vi "picoharp_start_stream.vi"(8 "error in (no error)":errorcluster, 11 "hydraharp in":refnum<class "picoharp.lvclass">) -> (0 "error out":errorcluster, 3 "hydraharp out":refnum<class "picoharp.lvclass">)   [LabVIEW 2015, in "picoharp.lvclass"]
uses:
  picoharp.lvclass
  picoharp.lvclass/picoharp.ctl
  Hydraharp/hydraharp/hydraharp_fifo_queue_data.ctl
  Hydraharp/hydraharp/hydraharp_fifo_actions.ctl
  Hydraharp/raw_stream_logger/raw_stream_logger.lvclass
  Hydraharp/hdf5_photon_record_logger/hdf5_photon_record_log.lvclass
  Data Logger Class/data_logger.lvclass
  phlib.dll
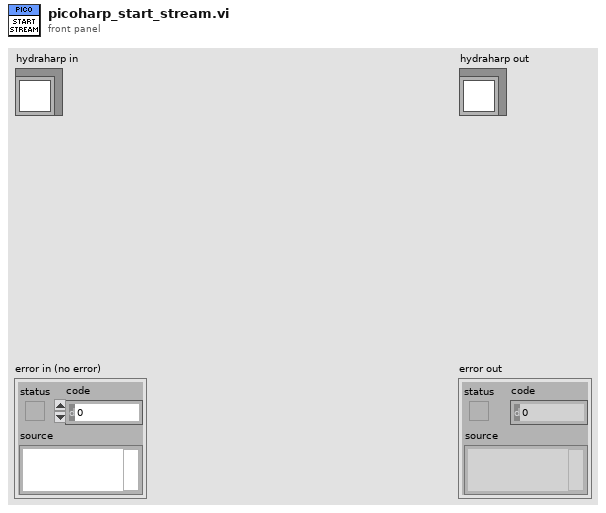
[diagram p1: front panel]
types:
  T1 = typedef "hydraharp_fifo_queue_data.ctl" = cluster{"fifo_buffer":u32[], "fifo_action":T2}
  T2 = typedef "hydraharp_fifo_actions.ctl" = enum16{"stop", "new_data"}
  T3 = typedef "hydraharp_action_on_records.ctl" = enum16{"stream_to_file", "correlate", "stream to file and correlate"}
  T4 = typedef "hpanel_acq_modes.ctl" = u16
  T5 = typedef "record_type.ctl" = enum16{"Raw Stream", "Processed Records (hdf5)"}
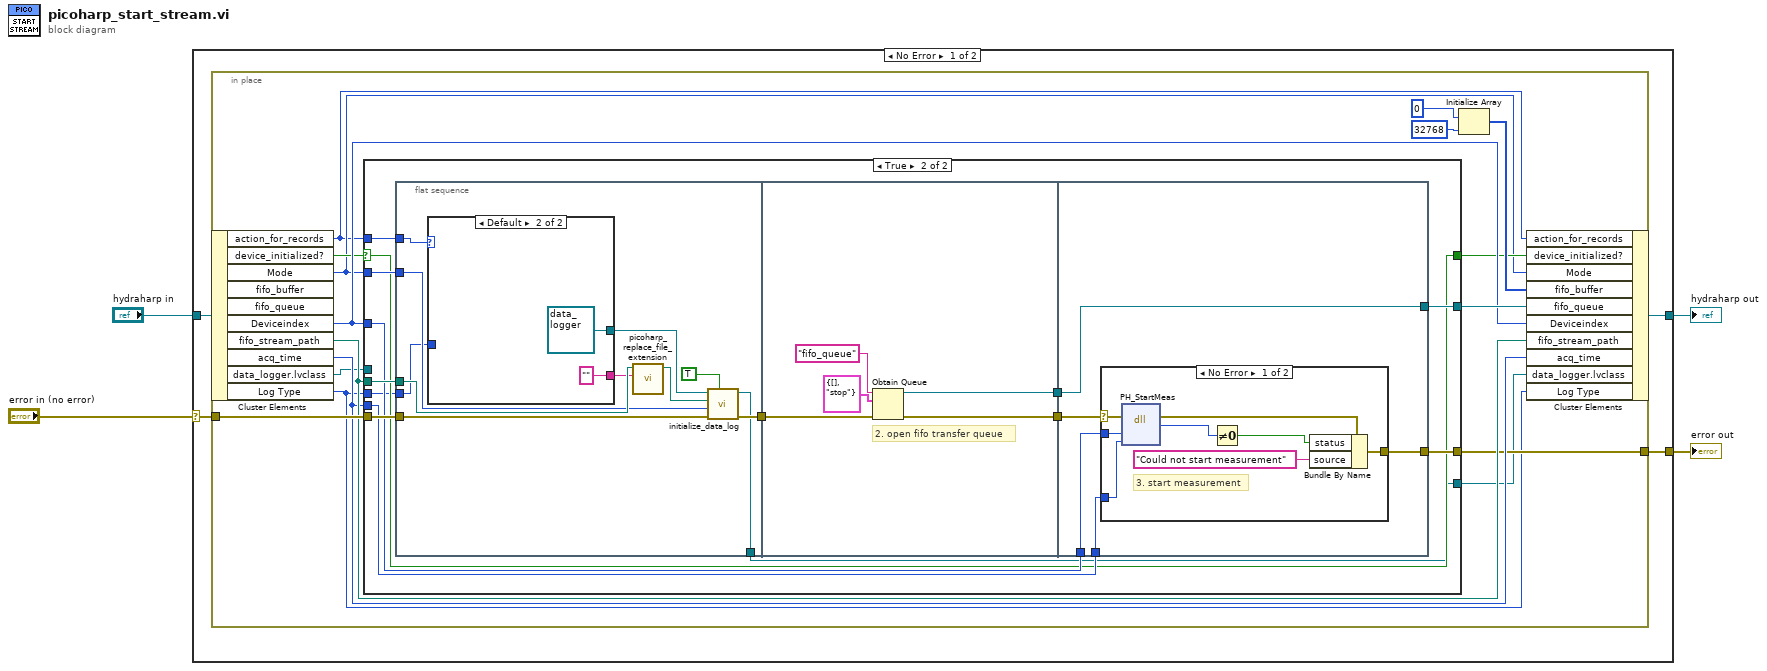
[diagram p0: block diagram]
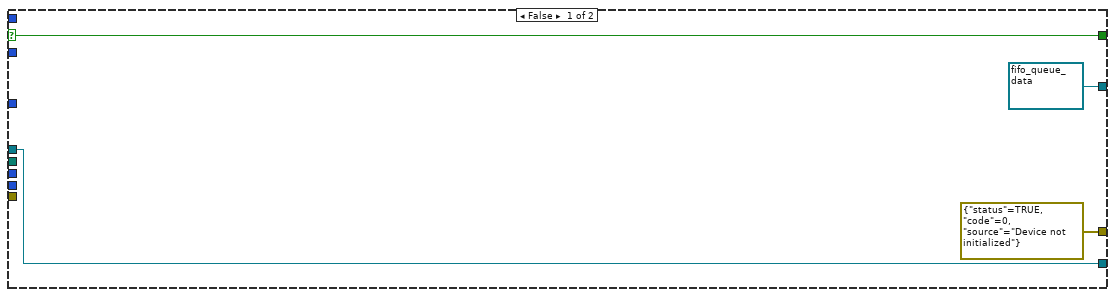
[diagram p2: hidden frame]
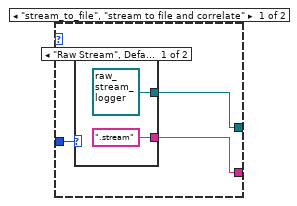
[diagram p3: hidden frame]
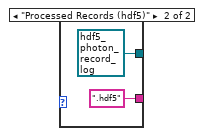
[diagram p4: hidden frame]
diagram:
  n1 = case shown="No Error" "error in (no error)" {
    selector: "error in (no error)" -> [w7 w83]
    tunnel: [w5 w83] -> w3
    tunnel: [w6 w82] -> w1
    tunnel: "hydraharp in" -> [w8 w82]
    frame No Error {
      n2 = in-place {
        in-place-border: w7 -> [w21]
        in-place-border: [w17] -> w5
        n3 = in-place-cluster #1(w8) -> ("action_for_records"=w10:T3, "device_initialized?"=w15:bool, "Mode"=w13:T4, "Deviceindex"=w16:i32, "fifo_stream_path"=w20:path, "acq_time"=w18:i32, "data_logger.lvclass"=w11:refnum<class "data_logger.lvclass">, "Log Type"=w9:T5)  [unwired: 2 out]
        n4 = case shown="True" w15 {
          selector: w15 -> [w26 w33]
          tunnel: w21 -> [_ w40]
          tunnel: w20 -> [_ w39]
          tunnel: [refnum<queue> refnum ("queue out") w38] -> w19
          tunnel: w18 -> [_ w37]
          tunnel: [errorcluster {"status"=TRUE, "code"=0, "source"="Device not initialized"} ("error IO") w36] -> w17
          tunnel: w16 -> [_ w35]
          tunnel: w13 -> [_ w34]
          tunnel: [w26 w33] -> w14
          tunnel: [w25 w31] -> w12
          tunnel: w11 -> [w25 _]
          tunnel: w10 -> [_ w30]
          tunnel: w9 -> [_ w29]
          frame False {
          }
          frame True {
            n5 = flat-sequence {
              tunnel: w40 -> [w50]
              tunnel: w39 -> [w53]
              tunnel: [w51] -> w32
              tunnel: w34 -> [w52]
              tunnel: [w49] -> w31
              tunnel: w30 -> [w45]
              tunnel: w29 -> [w44]
              tunnel: [w64] -> w42
              tunnel: [w63] -> w41
              tunnel: w32 -> [w65]
              tunnel: [w72] -> w38
              tunnel: w42 -> [w68]
              tunnel: w41 -> [w72]
              tunnel: w37 -> [w71]
              tunnel: [w70] -> w36
              tunnel: w35 -> [w69]
              frame #0 {
                n6 = case shown="Default" w45 {
                  tunnel: [w56 refnum<class "data_logger.lvclass"> refnum ("data_logger.lvclass")] -> w47
                  tunnel: w44 -> [w55 _]
                  tunnel: [w54 "" ("new_extension")] -> w43
                  frame "stream_to_file", "stream to file and correlate" {
                    n7 = case shown="\"Raw Stream\", Default" w55 {
                      tunnel: [refnum<class "raw_stream_logger.lvclass"> refnum ("raw_stream_logger.lvclass") refnum<class "hdf5_photon_record_log.lvclass"> refnum ("hdf5_photon_record_log.lvclass")] -> w56
                      tunnel: [".stream" ("new_extension") ".hdf5" ("new_extension")] -> w54
                      frame "Raw Stream", Default {
                      }
                      frame "Processed Records (hdf5)" {
                      }
                    }
                  }
                  frame Default {
                  }
                }
                n8 = call "picoharp_replace_file_extension.vi"("new_extension"=w43, "input_file"=w53) -> ("new_name"=w46:path)  [unwired: 9 in]
                n9 = call-dynamic "initialize_data_log.vi"("Overwrite?"=TRUE, "error in (no error)"=w50, "Initialization Data"=w52, "Path"=w46, "data_logger in"=w47) -> ("error out"=w51:errorcluster, "data_logger out"=w49:refnum<class "data_logger.lvclass">)  [unwired: 5 in]
              }
              frame #1 {
                # "2. open fifo transfer queue"
                n10 = Obtain Queue(name (unnamed)="fifo_queue", element data type=T1 {"fifo_buffer"=[], "fifo_action"=enum."stop"} ("fifo_queue_data"), error in (no error)=w65) -> (queue out=w63:refnum<queue>, error out=w64:errorcluster)  [unwired: 2 in, 1 out]
              }
              frame #2 {
                n11 = case shown="No Error" w68 {
                  selector: w68 -> [w73 w81]
                  tunnel: w71 -> [w80 _]
                  tunnel: [w75 w81] -> w70
                  tunnel: w69 -> [w74 _]
                  frame No Error {
                    # "3. start measurement"
                    n12 = dll-call lib="phlib.dll" fn="PH_StartMeas" label="pH_StartMeas"(error in=w73, "devidx"=w74, "tacq"=w80) -> (error out=w78:errorcluster, "return type"=w79:i32)  [unwired: 4 in, 1 out]
                    n13 = Not Equal To 0?(x=w79) -> (x != 0?=w77:bool)
                    n14 = Bundle By Name(cluster=w78, "status"=w77, "source"="Could not start measurement") -> (w75:errorcluster)
                  }
                  frame Error {
                  }
                }
              }
            }
          }
        }
        n15 = Initialize Array(u32 0 ("element"), 32768 ("dimension size")) -> (w24:u32[])
        n16 = in-place-cluster #1("action_for_records"=w10, "device_initialized?"=w14, "Mode"=w13, "fifo_buffer"=w24, "fifo_queue"=w19, "Deviceindex"=w16, "fifo_stream_path"=w20, "acq_time"=w18, "data_logger.lvclass"=w12, "Log Type"=w9) -> (w6:refnum<class "picoharp.lvclass">)
      }
    }
    frame Error {
    }
  }
  "error out" <- w3
  "hydraharp out" <- w1
